vi "dvp Vi Get Strobe Duration.vi"(10 "pStrobeDuration":dbl, 11 "handle":u32) -> (2 "pStrobeDuration out":dbl, 3 "function return":u32(ring))   [LabVIEW 2018, in "LabViewDVPCamera.lvlib"]
doc: "LabviewDvp2Api dvpStatus dvpViGetStrobeDuration(dvpHandle handle, double *pStrobeDuration);"
uses:
  LabViewDVPCamera.lvlib
  LabViewDVPCamera/LabViewDVPCamera.dll
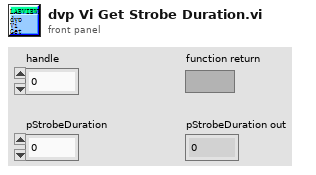
[diagram p1: front panel]
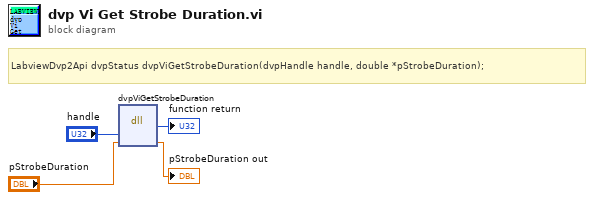
[diagram p0: block diagram]
diagram:
  # "LabviewDvp2Api dvpStatus dvpViGetStrobeDuration(dvpHandle handle, double *pStrobeDuration);"
  n1 = dll-call lib="C:/Program Files (x86)/DVP2 Labview cn 64/Sample/LabViewDVPCamera/LabViewDVPCamera.*" fn="dvpViGetStrobeDuration"("handle"="handle", "pStrobeDuration"="pStrobeDuration") -> (→"function return":u32, "pStrobeDuration"=→"pStrobeDuration out":dbl)  [unwired: 4 in, 2 out]
